vi "Turn on point PID.vi"(4 "Range":cluster{"output high":dbl, "output low":dbl}={"output high"=1.0, "output low"=-1.0} {"output low" format="%.2f"; "output high" format="%.2f"}, 5 "Loop Timer":i32=20, 6 "Gains":T1={"proportional gain (Kc)"=1.0, "integral time (Ti, min)"=0.01, "derivative time (Td, min)"=0.0} {"derivative time (Td, min)" format="%.3f"; "integral time (Ti, min)" format="%.3f"; "proportional gain (Kc)" format="%.3f"}, 7 "Time to stop":i32=300, 8 "Precision":dbl=0.5 format="%#_13g", 10 "Yaw":dbl, 11 "Setpoint(degrees)":dbl=90.0) -> (0 "Finished?":bool, 2 "PWM right":dbl, 3 "PWM left":dbl)   [LabVIEW 2017]
panel:
  # "Time to stop - Tempo que o encoder deve retornar um valor dentro do range da precision para a função considerar que o sistema está parado.\n\nSetpoint- Setpoint em graus\n\nLoop Timer - Tempo de iteração do loop em que a função está.\n\nPrecision - Range que a função considera \"close enough\" ao setpoint.\n\nYaw - Valor atual do NavX.\n\nGains - Ganhos do PID.\n\nRange - limite superior e inferior do PID."
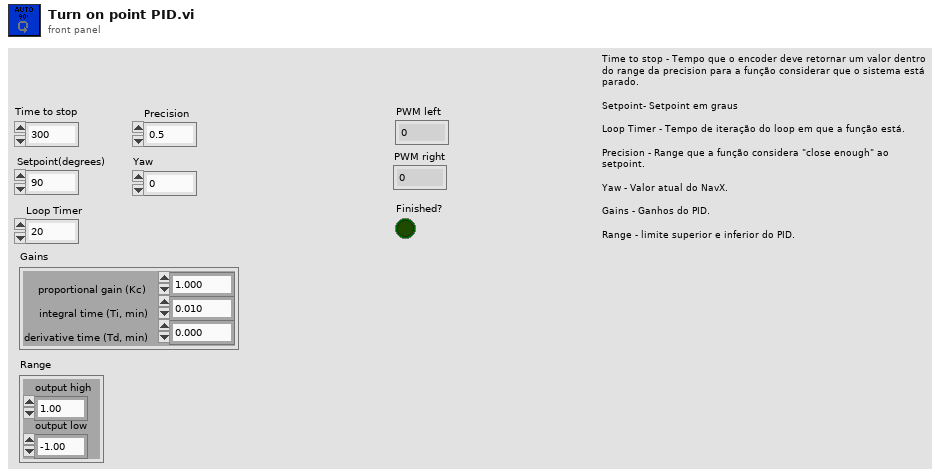
[diagram p1: front panel]
types:
  T1 = cluster{"proportional gain (Kc)":dbl, "integral time (Ti, min)":dbl, "derivative time (Td, min)":dbl}
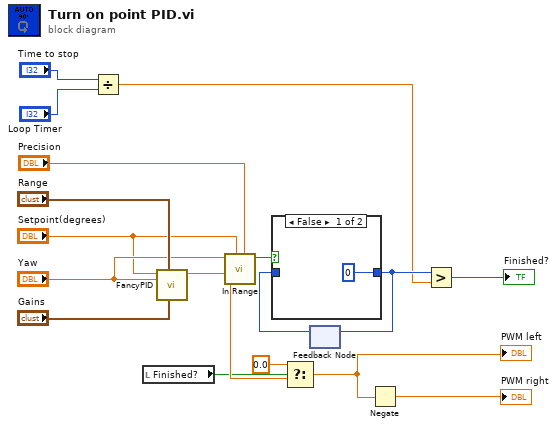
[diagram p0: block diagram]
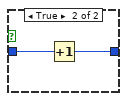
[diagram p2: hidden frame]
diagram:
  n1 = Divide(x="Time to stop", y="Loop Timer") -> (x/y=w14:dbl)
  n2 = local read "Finished?"() -> (w1:bool)
  n3 = call "FancyPID.vi"("Gains"="Gains", "Range"="Range", "Process variable"="Yaw", "Setpoint"="Setpoint(degrees)") -> ("output"=w3:dbl)  [unwired: 7 in]
  n4 = call "In Range.vi"("Range"="Precision", "Setpoint"="Setpoint(degrees)", "Value"="Yaw") -> ("in range?"=w6:bool)  [unwired: 8 in]
  n5 = Select(t=0.0, s=w1, f=w3) -> (s? t:f=w4:dbl)
  "PWM left" <- w4
  n6 = feedback #1() -> (w16:i32)  [unwired: 1 in]
  n7 = case shown="False" w6 {
    tunnel: [0 w20] -> w15
    tunnel: w16 -> [_ w19]
    frame False {
    }
    frame True {
      n8 = Increment(x=w19) -> (x+1=w20:i32)
    }
  }
  n9 = feedback-in #1(w15) -> ()
  n10 = Negate(x=w4) -> (-x=→"PWM right":dbl)
  n11 = Greater?(x=w15, y=w14) -> (0:→"Finished?":bool)
